vi "WLAN - TV - CreateTestVectors.vi"() -> ()   [LabVIEW 2011]
uses:
  RW/Includes/WLAN - TV - RW - INC - TV_IQComposite_11A.ctl
  RW/Includes/WLAN - TV - RW - INC - TV_OFDM Demod.ctl
  RW/Includes/WLAN - TV - RW - INC - TV_IQComposite_11B.ctl
  RW/Includes/WLAN - TV - RW - INC - TV_DSSS Demod.ctl
  RW/Includes/WLAN - TV - RW - INC - TV_IQComposite_11N.ctl
  RW/Includes/WLAN - TV - RW - INC - TV_IQComposite_11AC.ctl
  RW/Includes/WLAN - TV - RW - INC - Select TV to Generate.ctl
  RW/Includes/WLAN - TV - RW - INC - TV_Parameters.ctl
  <vilib>/Utility/file.llb/Write To Spreadsheet File (string).vi
  <vilib>/Utility/file.llb/Write To Spreadsheet File (DBL).vi
panel:
  in  "TV Paramaters":T1
  in  "Measurement Type 802.11G 5":enum32{"Tx Measurement", "Rx Measurement "}(tab)
  in  "Standard":T2(tab)=enum."802.11A/G(OFDM)"
  in  "Select TV":T3={"Tx_ 802.11a/g OFDM"=TRUE, "Tx_ 802.11b DSSS/CCK"=TRUE, "Tx_ 802.11n OFDM "=TRUE, "Tx_ 802.11ac OFDM "=FALSE}
  in  "TV_Tx_11A/G OFDM":T4={"Standard"=0, "Generation Parameters"=[{"Power Level(dBm)"=[15.0], "Center Frequency(Hz)"=[2412000000.0, 5180000000.0, 5700000000.0], "Payload Control"=[{"OFDM Data Rate (Mbps)"=3, "OFDM Payload Length (bytes)"=200, "Idle Interval (s)"=0.0001}, {"OFDM Data Rate (Mbps)"=7, "OFDM Payload Length (bytes)"=600, "Idle Interval (s)"=0.0001}]}], "OFDM Advanced Controls"={"OFDM Auto Compute Acquisition Length Enabled"=1, "OFDM Maximum Symbols Used"=16, "OFDM Time Tracking Enabled"=1, "OFDM Channel Tracking Enabled"=0, "OFDM Amplitude Tracking Enabled"=0, "OFDM CFO Estimation Method"=0, "OFDM Phase Tracking Method"=0, "OFDM Header Detection Enabled"=0, "OFDM MAC FCS Check Enabled"=0, "#Avg"=3, "#Iterations"=1}, "Measurement  Enabled ?"=TRUE, "#Packets"=0} {"OFDM Advanced Controls"."OFDM Phase Tracking Method" items=["Standard", "Instantaneous", "None", "Standard with Cubic Spline Fit"]; "OFDM Advanced Controls"."OFDM CFO Estimation Method" items=["Preamble Only", "Preamble and Data"]; "OFDM Advanced Controls"."OFDM Channel Tracking Enabled" items=["False", "True"]; "OFDM Advanced Controls"."OFDM Amplitude Tracking Enabled" items=["False", "True"]; "OFDM Advanced Controls"."OFDM Time Tracking Enabled" items=["True"=1, "False"=0]; "OFDM Advanced Controls"."OFDM Auto Compute Acquisition Length Enabled" items=["False", "True"]; "OFDM Advanced Controls"."OFDM MAC FCS Check Enabled" items=["False", "True"]; "OFDM Advanced Controls"."OFDM Header Detection Enabled" items=["False", "True"]; "Generation Parameters"."Payload Control"."OFDM Data Rate (Mbps)" items=["6", "9", "12", "18", "24", "36", "48", "54"]; "Generation Parameters"."Center Frequency(Hz)" format="%#_6p"; "Standard" items=["80211A/G/J/P OFDM", "80211B/G DSSS", "80211G DSSSOFDM", "80211N MIMOOFDM", "80211AC MIMOOFDM"]}
  in  "TV_TX_80211B":T6={"Standard"=1, "DSSS Demod Parameters"={"DSSS Auto Compute Acquisition Length Enabled"=1, "DSSS Equalization Enabled"=0, "DSSS Header Detection Enabled"=0, "DSSS MAC FCS Check Enabled"=0, "DSSS Measurement Start Location"=0, "DSSS Phase Tracking Method"=0, "DSSS Maximum Chips Used"=1000, "DSSS Reference Pulse Shaping Filter"=3, "DSSS Reference Pulse Shaping Filter Coefficient"=0.4, "# Avg"=3, "# Iterations"=1, "DSSS Power Ramp Enabled"=1}, "DSSS Gen Paramaters"=[{"Generation Properties"=[{"DSSS Data Rate (Mbps)"=0, "DSSS Payload Length (bytes)"=10, "Idle Interval(S)"=0.00025}, {"DSSS Data Rate (Mbps)"=4, "DSSS Payload Length (bytes)"=100, "Idle Interval(S)"=0.00025}], "Power Level(dBm)"=[15.0], "Center Frequency(Hz)"=[2412000000.0, 2432000000.0]}], "Measurement Enabled ? "=TRUE} {"DSSS Gen Paramaters"."Center Frequency(Hz)" format="%#_6p"; "DSSS Gen Paramaters"."Generation Properties"."DSSS Data Rate (Mbps)" items=["1", "2", "5.5 CCK", "5.5 PBCC", "11 CCK", "11 PBCC", "22", "33"]; "DSSS Demod Parameters"."DSSS Power Ramp Enabled" items=["False", "True"]; "DSSS Demod Parameters"."DSSS Auto Compute Acquisition Length Enabled" items=["False", "True"]; "DSSS Demod Parameters"."DSSS Phase Tracking Method" items=["Standard", "Instantaneous"]; "DSSS Demod Parameters"."DSSS Equalization Enabled" items=["False", "True"]; "DSSS Demod Parameters"."DSSS Reference Pulse Shaping Filter" items=["Rectangular", "Raised Cosine", "Root Raised Cosine", "Gaussian"]; "DSSS Demod Parameters"."DSSS MAC FCS Check Enabled" items=["False", "True"]; "DSSS Demod Parameters"."DSSS Header Detection Enabled" items=["False", "True"]; "Standard" items=["80211A/G/J/P OFDM", "80211B/G DSSS", "80211G DSSSOFDM", "80211N MIMOOFDM", "80211AC MIMOOFDM"]}
  in  "TV_Tx_80211N":T8={"Standard"=3, "80211n PLCP Frame Format"=[0], "FEC Coding Type"=[0], "Guard Interval (s)"=[8e-07], "Measurment Settings"={"OFDM Auto Compute Acquisition Length Enabled"=1, "OFDM Maximum Symbols Used"=16, "OFDM Time Tracking Enabled"=1, "OFDM Channel Tracking Enabled"=0, "OFDM Amplitude Tracking Enabled"=0, "OFDM CFO Estimation Method"=0, "OFDM Phase Tracking Method"=0, "OFDM Header Detection Enabled"=0, "OFDM MAC FCS Check Enabled"=0, "#Avg"=3, "#Iterations"=1}, "Generation Parameters"=[{"Generation Parameters"=[{"Channel Bandwidth(Hz)"=20000000.0, "MCS Index"=4, "OFDM Payload Length (bytes)"=1024, "Idle Interval(S)"=0.0001}, {"Channel Bandwidth(Hz)"=20000000.0, "MCS Index"=7, "OFDM Payload Length (bytes)"=1024, "Idle Interval(S)"=0.0001}], "Center Frequency(Hz)"=[2412000000.0, 5180000000.0, 5700000000.0], "Power Level(dBm)"=[15.0]}], "Measurement Enabled"=TRUE, "#Packets"=0} {"Generation Parameters"."Center Frequency(Hz)" format="%#_6p"; "Generation Parameters"."Generation Parameters"."Channel Bandwidth(Hz)" items=["5M"=5000000.0, "10M"=10000000.0, "20M"=20000000.0, "40M"=40000000.0, "80M"=80000000.0, "160M"=160000000.0]; "Measurment Settings"."OFDM Phase Tracking Method" items=["Standard", "Instantaneous", "None", "Standard with Cubic Spline Fit"]; "Measurment Settings"."OFDM CFO Estimation Method" items=["Preamble Only", "Preamble and Data"]; "Measurment Settings"."OFDM Channel Tracking Enabled" items=["False", "True"]; "Measurment Settings"."OFDM Amplitude Tracking Enabled" items=["False", "True"]; "Measurment Settings"."OFDM Time Tracking Enabled" items=["True"=1, "False"=0]; "Measurment Settings"."OFDM Auto Compute Acquisition Length Enabled" items=["False", "True"]; "Measurment Settings"."OFDM MAC FCS Check Enabled" items=["False", "True"]; "Measurment Settings"."OFDM Header Detection Enabled" items=["False", "True"]; "FEC Coding Type" items=["BCC", "LDPC"]; "80211n PLCP Frame Format" items=["Mixed Format", "Greenfield Format"]; "Standard" items=["80211A/G/J/P OFDM", "80211B/G DSSS", "80211G DSSSOFDM", "80211N MIMOOFDM", "80211AC MIMOOFDM"]}
  in  "TV_IQComposite_11AC":T9={"Standard"=4, "FEC Coding Type"=[0], "Guard Interval (s)"=[8e-07], "OFDM Advanced Controls"={"OFDM Auto Compute Acquisition Length Enabled"=1, "OFDM Maximum Symbols Used"=16, "OFDM Time Tracking Enabled"=1, "OFDM Channel Tracking Enabled"=0, "OFDM Amplitude Tracking Enabled"=0, "OFDM CFO Estimation Method"=0, "OFDM Phase Tracking Method"=0, "OFDM Header Detection Enabled"=1, "OFDM MAC FCS Check Enabled"=0, "#Avg"=1, "#Iterations"=1}, "Generation Parameters"=[{"Generation Parameters"=[{"Channel BW(Hz)"=40000000.0, "MCS Index"=0, "OFDM Payload Length (bytes)"=1600, "Idle Interval(S)"=0.0002, "N_SS"=3}, {"Channel BW(Hz)"=40000000.0, "MCS Index"=5, "OFDM Payload Length (bytes)"=1600, "Idle Interval(S)"=0.0002, "N_SS"=3}], "Center Frequency(Hz)"=[5190000000.0, 5270000000.0, 5510000000.0], "Power Level(dBm)"=[14.0, 12.0, 10.0]}, {"Generation Parameters"=[{"Channel BW(Hz)"=80000000.0, "MCS Index"=3, "OFDM Payload Length (bytes)"=1600, "Idle Interval(S)"=0.0002, "N_SS"=3}, {"Channel BW(Hz)"=80000000.0, "MCS Index"=5, "OFDM Payload Length (bytes)"=1600, "Idle Interval(S)"=0.0002, "N_SS"=3}, {"Channel BW(Hz)"=80000000.0, "MCS Index"=7, "OFDM Payload Length (bytes)"=1600, "Idle Interval(S)"=0.0002, "N_SS"=3}], "Center Frequency(Hz)"=[5210000000.0, 5290000000.0, 5530000000.0], "Power Level(dBm)"=[14.0, 12.0, 10.0]}], "Measurement Enabled"=TRUE, "#Packets"=0} {"Generation Parameters"."Center Frequency(Hz)" format="%#_6p"; "Generation Parameters"."Generation Parameters"."Channel BW(Hz)" items=["5M"=5000000.0, "10M"=10000000.0, "20M"=20000000.0, "40M"=40000000.0, "80M"=80000000.0, "160M"=160000000.0]; "OFDM Advanced Controls"."OFDM Phase Tracking Method" items=["Standard", "Instantaneous", "None", "Standard with Cubic Spline Fit"]; "OFDM Advanced Controls"."OFDM CFO Estimation Method" items=["Preamble Only", "Preamble and Data"]; "OFDM Advanced Controls"."OFDM Channel Tracking Enabled" items=["False", "True"]; "OFDM Advanced Controls"."OFDM Amplitude Tracking Enabled" items=["False", "True"]; "OFDM Advanced Controls"."OFDM Time Tracking Enabled" items=["True"=1, "False"=0]; "OFDM Advanced Controls"."OFDM Auto Compute Acquisition Length Enabled" items=["False", "True"]; "OFDM Advanced Controls"."OFDM MAC FCS Check Enabled" items=["False", "True"]; "OFDM Advanced Controls"."OFDM Header Detection Enabled" items=["False", "True"]; "FEC Coding Type" items=["BCC", "LDPC"]; "Standard" items=["80211A/G/J/P OFDM", "80211B/G DSSS", "80211G DSSSOFDM", "80211N MIMOOFDM", "80211AC MIMOOFDM"]}
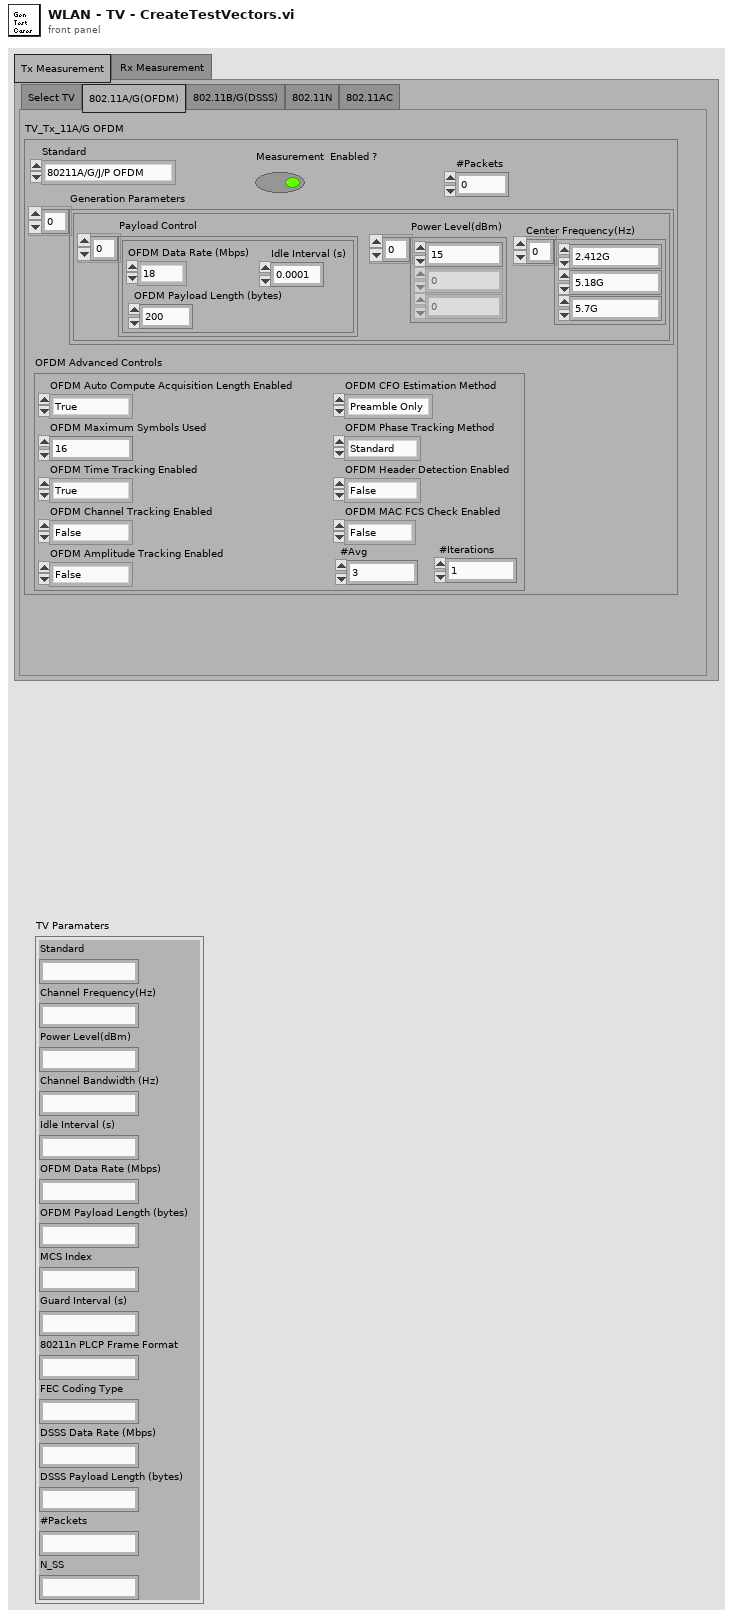
[diagram p1: front panel]
types:
  T1 = typedef "WLAN - TV - RW - INC - TV_Parameters.ctl" = cluster{"Standard ":string, "Channel Frequency(Hz)":string, "Power Level(dBm)":string, "Channel Bandwidth (Hz)":string, "Idle Interval (s)":string, "OFDM Data Rate (Mbps)":string, "OFDM Payload Length (bytes)":string, "MCS Index":string, "Guard Interval (s)":string, "80211n PLCP Frame Format":string, "FEC Coding Type":string, "DSSS Data Rate (Mbps)":string, "DSSS Payload Length (bytes)":string, "#Packets":string, "N_SS":string}
  T2 = enum32{"Select TV", "802.11A/G(OFDM)", "802.11B/G(DSSS)", "802.11N", "802.11AC"}
  T3 = typedef "WLAN - TV - RW - INC - Select TV to Generate.ctl" = cluster{"Tx_ 802.11a/g OFDM":bool, "Tx_ 802.11b DSSS/CCK":bool, "Tx_ 802.11n OFDM ":bool, "Tx_ 802.11ac OFDM ":bool}
  T4 = typedef "WLAN - TV - RW - INC - TV_IQComposite_11A.ctl" = cluster{"Standard":i32, "Generation Parameters":cluster{"Power Level(dBm)":dbl[], "Center Frequency(Hz)":dbl[], "Payload Control":cluster{"OFDM Data Rate (Mbps)":i32, "OFDM Payload Length (bytes)":i32, "Idle Interval (s)":dbl}[]}[], "OFDM Advanced Controls":T5, "Measurement  Enabled ?":bool, "#Packets":i32}
  T5 = typedef "WLAN - TV - RW - INC - TV_OFDM Demod.ctl" = cluster{"OFDM Auto Compute Acquisition Length Enabled":i32, "OFDM Maximum Symbols Used":i32, "OFDM Time Tracking Enabled":i32, "OFDM Channel Tracking Enabled":i32, "OFDM Amplitude Tracking Enabled":i32, "OFDM CFO Estimation Method":i32, "OFDM Phase Tracking Method":i32, "OFDM Header Detection Enabled":i32, "OFDM MAC FCS Check Enabled":i32, "#Avg":i32, "#Iterations":i32}
  T6 = typedef "WLAN - TV - RW - INC - TV_IQComposite_11B.ctl" = cluster{"Standard":i32, "DSSS Demod Parameters":T7, "DSSS Gen Paramaters":cluster{"Generation Properties":cluster{"DSSS Data Rate (Mbps)":i32, "DSSS Payload Length (bytes)":i32, "Idle Interval(S)":dbl}[], "Power Level(dBm)":dbl[], "Center Frequency(Hz)":dbl[]}[], "Measurement Enabled ? ":bool}
  T7 = typedef "WLAN - TV - RW - INC - TV_DSSS Demod.ctl" = cluster{"DSSS Auto Compute Acquisition Length Enabled":i32, "DSSS Equalization Enabled":i32, "DSSS Header Detection Enabled":i32, "DSSS MAC FCS Check Enabled":i32, "DSSS Measurement Start Location":i32, "DSSS Phase Tracking Method":i32, "DSSS Maximum Chips Used":i32, "DSSS Reference Pulse Shaping Filter":i32, "DSSS Reference Pulse Shaping Filter Coefficient":dbl, "# Avg":i32, "# Iterations":i32, "DSSS Power Ramp Enabled":i32}
  T8 = typedef "WLAN - TV - RW - INC - TV_IQComposite_11N.ctl" = cluster{"Standard":i32, "80211n PLCP Frame Format":i32[], "FEC Coding Type":i32[], "Guard Interval (s)":dbl[], "Measurment Settings":T5, "Generation Parameters":cluster{"Generation Parameters":cluster{"Channel Bandwidth(Hz)":dbl, "MCS Index":i32, "OFDM Payload Length (bytes)":i32, "Idle Interval(S)":dbl}[], "Center Frequency(Hz)":dbl[], "Power Level(dBm)":dbl[]}[], "Measurement Enabled":bool, "#Packets":i32}
  T9 = typedef "WLAN - TV - RW - INC - TV_IQComposite_11AC.ctl" = cluster{"Standard":i32, "FEC Coding Type":i32[], "Guard Interval (s)":dbl[], "OFDM Advanced Controls":T5, "Generation Parameters":cluster{"Generation Parameters":cluster{"Channel BW(Hz)":dbl, "MCS Index":i32, "OFDM Payload Length (bytes)":i32, "Idle Interval(S)":dbl, "N_SS":i32}[], "Center Frequency(Hz)":dbl[], "Power Level(dBm)":dbl[]}[], "Measurement Enabled":bool, "#Packets":i32}
  T10 = cluster{"TV_Tx_11A/G OFDM":T4, "TV_TX_80211B":T6, "TV_Tx_80211N ":T8, "TV_IQComposite_11AC":T9}
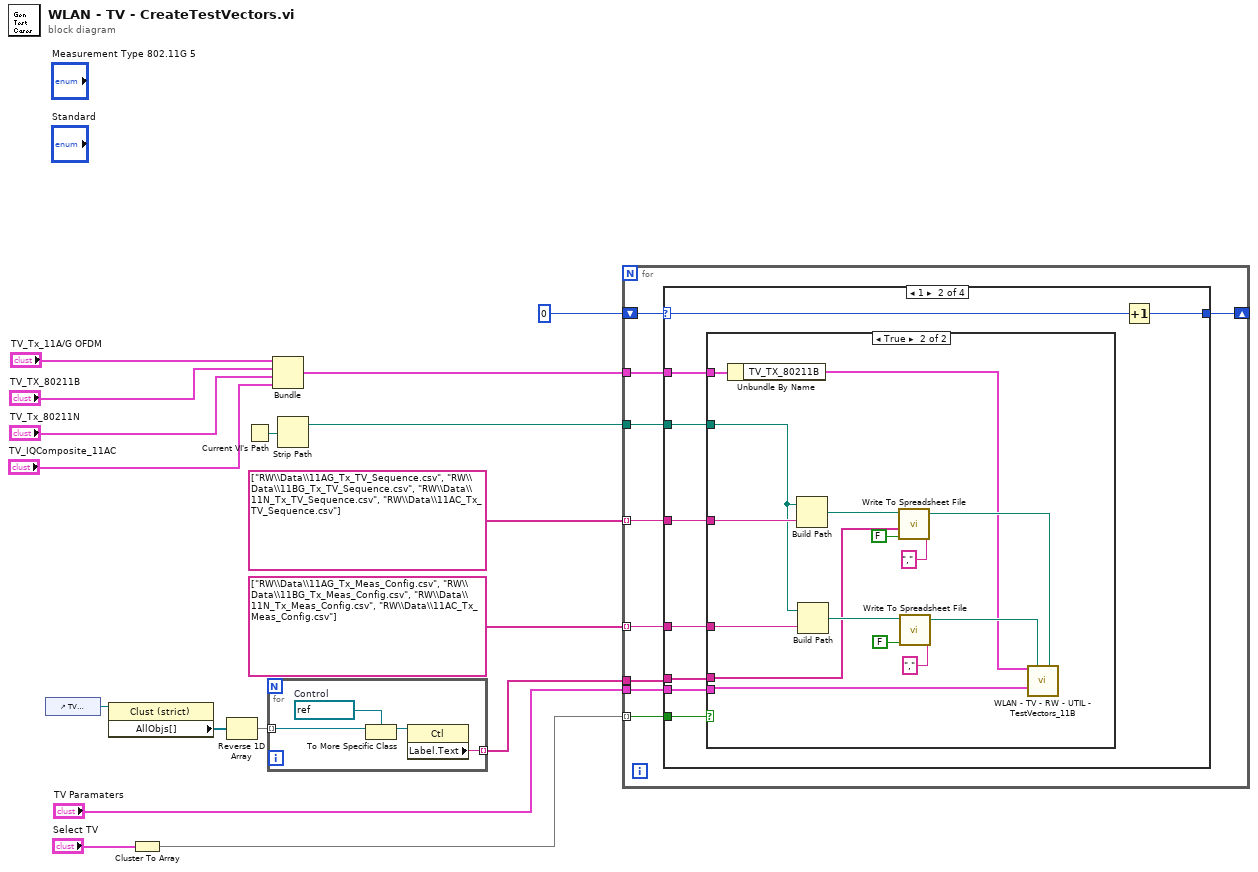
[diagram p0: block diagram]
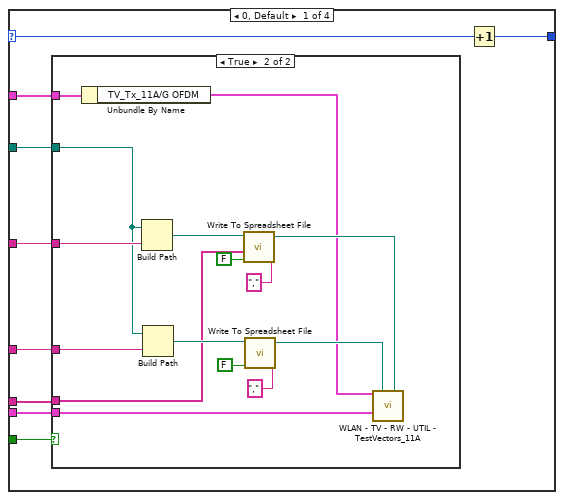
[diagram p2: hidden frame]
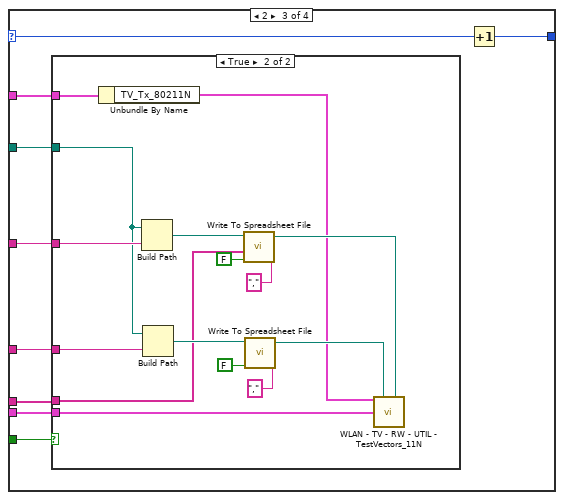
[diagram p5: hidden frame]
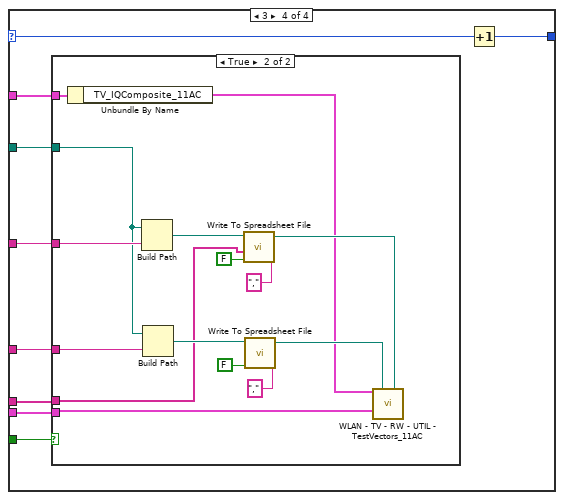
[diagram p7: hidden frame]
diagram:
  n1 = control-ref of="TV Paramaters"() -> (w3:refnum<vi>)
  n2 = property class="Clust (strict)"(reference=w3) -> ("AllObjs[]"=w4:refnum<vi>[])  [unwired: 1 in, 2 out]
  n3 = Cluster To Array(cluster="Select TV") -> (array=w13:bool[])
  n4 = Reverse 1D Array(array=w4) -> (reversed array=w1:refnum<vi>[])
  n5 = Current VI's Path() -> (path=w17:path)
  n6 = for {
    tunnel: w1 -> [w20] mode=indexing
    tunnel: [w21] -> w2 mode=indexing
    w19 = refnum<vi> refnum  # Control
    n7 = To More Specific Class(target class=w19, reference=w20) -> (specific class reference=w18:refnum<vi>)  [unwired: 1 in, 1 out]
    n8 = property class="Ctl"(reference=w18) -> ("Label.Text"=w21:string)  [unwired: 1 in, 2 out]
  }
  n9 = Bundle("TV_Tx_11A/G OFDM"="TV_Tx_11A/G OFDM", "TV_TX_80211B"="TV_TX_80211B", "TV_Tx_80211N"="TV_Tx_80211N", "TV_IQComposite_11AC"="TV_IQComposite_11AC") -> (w6:T10)  [unwired: 1 in]
  n10 = Strip Path(path=w17) -> (stripped path=w11:path)  [unwired: 1 out]
  n11 = for {
    tunnel: string[] ["RW\\Data\\11AG_Tx_TV_Sequence.csv", "RW\\Data\\11BG_Tx_TV_Sequence.csv", "RW\\Data\\11N_Tx_TV_Sequence.csv", "RW\\Data\\11AC_Tx_TV_Sequence.csv"] -> [w26] mode=indexing
    tunnel: string[] ["RW\\Data\\11AG_Tx_Meas_Config.csv", "RW\\Data\\11BG_Tx_Meas_Config.csv", "RW\\Data\\11N_Tx_Meas_Config.csv", "RW\\Data\\11AC_Tx_Meas_Config.csv"] -> [w27] mode=indexing
    tunnel: w13 -> [w30] mode=indexing
    shift-right: [w28] -> _
    shift-left: 0 -> [w29]
    tunnel: w11 -> [w25]
    tunnel: w2 -> [w24]
    tunnel: w6 -> [w23]
    tunnel: "TV Paramaters" -> [w22]
    n12 = case shown="1" w29 {
      selector: w29 -> [w38 w62 w86 w110]
      tunnel: w30 -> [w39 w63 w87 w111]
      tunnel: [w37 w61 w85 w109] -> w28
      tunnel: w27 -> [w36 w60 w84 w108]
      tunnel: w26 -> [w35 w59 w83 w107]
      tunnel: w25 -> [w34 w58 w82 w106]
      tunnel: w24 -> [w33 w57 w81 w105]
      tunnel: w23 -> [w32 w56 w80 w104]
      tunnel: w22 -> [w31 w55 w79 w103]
      frame 0, Default {
        n13 = case shown="True" w39 {
          tunnel: w36 -> [_ w48]
          tunnel: w35 -> [_ w47]
          tunnel: w34 -> [_ w46]
          tunnel: w33 -> [_ w40]
          tunnel: w32 -> [_ w43]
          tunnel: w31 -> [_ w41]
          frame False {
          }
          frame True {
            n14 = Unbundle By Name(w43) -> ("TV_Tx_11A/G OFDM"=w42:T4)
            n15 = Build Path(base path=w46, name or relative path=w47) -> (appended path=w52:path)
            n16 = Build Path(base path=w46, name or relative path=w48) -> (appended path=w53:path)
            n17 = call-poly <vilib>:"Write To Spreadsheet File.vi"("delimiter (\\t)"="," ("delimiter (\\t)"), "append to file? (new file:F)"=FALSE, "1D data"=w40, "file path (dialog if empty)"=w52) -> ("new file path (Not A Path if cancelled)"=w45:path)  [unwired: 4 in]
            n18 = call-poly <vilib>:"Write To Spreadsheet File.vi"("delimiter (\\t)"="," ("delimiter (\\t)"), "append to file? (new file:F)"=FALSE, "file path (dialog if empty)"=w53) -> ("new file path (Not A Path if cancelled)"=w44:path)  [unwired: 5 in]
            n19 = call "WLAN - TV - RW - UTIL - TestVectors_11A.vi"("TV_IQComposite_11A"=w42, "11a_Meas_Config"=w44, "TV_802_11a"=w45, "TV Paramaters"=w41) -> ()  [unwired: 12 in]
          }
        }
        n20 = Increment(x=w38) -> (x+1=w37:i32)
      }
      frame 1 {
        n21 = case shown="True" w63 {
          tunnel: w60 -> [_ w72]
          tunnel: w59 -> [_ w71]
          tunnel: w58 -> [_ w70]
          tunnel: w57 -> [_ w65]
          tunnel: w56 -> [_ w67]
          tunnel: w55 -> [_ w64]
          frame False {
          }
          frame True {
            n22 = Unbundle By Name(w67) -> ("TV_TX_80211B"=w66:T6)
            n23 = Build Path(base path=w70, name or relative path=w71) -> (appended path=w76:path)
            n24 = Build Path(base path=w70, name or relative path=w72) -> (appended path=w77:path)
            n25 = call-poly <vilib>:"Write To Spreadsheet File.vi"("delimiter (\\t)"="," ("delimiter (\\t)"), "append to file? (new file:F)"=FALSE, "1D data"=w65, "file path (dialog if empty)"=w76) -> ("new file path (Not A Path if cancelled)"=w69:path)  [unwired: 4 in]
            n26 = call-poly <vilib>:"Write To Spreadsheet File.vi"("delimiter (\\t)"="," ("delimiter (\\t)"), "append to file? (new file:F)"=FALSE, "file path (dialog if empty)"=w77) -> ("new file path (Not A Path if cancelled)"=w68:path)  [unwired: 5 in]
            n27 = call "WLAN - TV - RW - UTIL - TestVectors_11B.vi"("TV_IQComposite_11B"=w66, "11b_Meas_Config"=w68, "TV_802_11b"=w69, "TV Paramaters"=w64) -> ()  [unwired: 12 in]
          }
        }
        n28 = Increment(x=w62) -> (x+1=w61:i32)
      }
      frame 2 {
        n29 = case shown="True" w87 {
          tunnel: w84 -> [_ w96]
          tunnel: w83 -> [_ w95]
          tunnel: w82 -> [_ w94]
          tunnel: w81 -> [_ w89]
          tunnel: w80 -> [_ w91]
          tunnel: w79 -> [_ w88]
          frame False {
          }
          frame True {
            n30 = Unbundle By Name(w91) -> ("TV_Tx_80211N"=w90:T8)
            n31 = Build Path(base path=w94, name or relative path=w95) -> (appended path=w100:path)
            n32 = Build Path(base path=w94, name or relative path=w96) -> (appended path=w101:path)
            n33 = call-poly <vilib>:"Write To Spreadsheet File.vi"("delimiter (\\t)"="," ("delimiter (\\t)"), "append to file? (new file:F)"=FALSE, "1D data"=w89, "file path (dialog if empty)"=w100) -> ("new file path (Not A Path if cancelled)"=w93:path)  [unwired: 4 in]
            n34 = call-poly <vilib>:"Write To Spreadsheet File.vi"("delimiter (\\t)"="," ("delimiter (\\t)"), "append to file? (new file:F)"=FALSE, "file path (dialog if empty)"=w101) -> ("new file path (Not A Path if cancelled)"=w92:path)  [unwired: 5 in]
            n35 = call "WLAN - TV - RW - UTIL - TestVectors_11N.vi"("TV_IQComposite_11N"=w90, "11n_Meas_Config"=w92, "TV_802_11n"=w93, "TV Paramaters"=w88) -> ()  [unwired: 12 in]
          }
        }
        n36 = Increment(x=w86) -> (x+1=w85:i32)
      }
      frame 3 {
        n37 = case shown="True" w111 {
          tunnel: w108 -> [_ w120]
          tunnel: w107 -> [_ w119]
          tunnel: w106 -> [_ w118]
          tunnel: w105 -> [_ w113]
          tunnel: w104 -> [_ w115]
          tunnel: w103 -> [_ w112]
          frame False {
          }
          frame True {
            n38 = Unbundle By Name(w115) -> ("TV_IQComposite_11AC"=w114:T9)
            n39 = Build Path(base path=w118, name or relative path=w119) -> (appended path=w124:path)
            n40 = Build Path(base path=w118, name or relative path=w120) -> (appended path=w125:path)
            n41 = call-poly <vilib>:"Write To Spreadsheet File.vi"("delimiter (\\t)"="," ("delimiter (\\t)"), "append to file? (new file:F)"=FALSE, "1D data"=w113, "file path (dialog if empty)"=w124) -> ("new file path (Not A Path if cancelled)"=w116:path)  [unwired: 4 in]
            n42 = call-poly <vilib>:"Write To Spreadsheet File.vi"("delimiter (\\t)"="," ("delimiter (\\t)"), "append to file? (new file:F)"=FALSE, "file path (dialog if empty)"=w125) -> ("new file path (Not A Path if cancelled)"=w117:path)  [unwired: 5 in]
            n43 = call "WLAN - TV - RW - UTIL - TestVectors_11AC.vi"("TV_IQComposite_11N"=w114, "11ac_Meas_Config"=w117, "TV_802_11ac"=w116, "TV Paramaters"=w112) -> ()  [unwired: 12 in]
          }
        }
        n44 = Increment(x=w110) -> (x+1=w109:i32)
      }
    }
  }
